vi "MQTT_Read_Published_Message.vi"(8 "error in (no error)":errorcluster, 11 "SSL_Connection":T2) -> (0 "error out":errorcluster, 1 "Message":string="MQIsdp", 2 "Topic Name":string="Topic", 3 "SSL_Connection":T2, 4 "MessageType":T1, 5 "Message ID":u16=1 format="%x")   [LabVIEW 2018, in "AWS_IoT.lvlib"]
doc: "This VI reads the last published message at the selected topic. It sends acknowledge information if required by the QoS level.\n\n© 2015 - daq.io, LLC - Peter Adelhardt"
uses:
  AWS_IoT.lvlib
  Controls/SSL_Connection.ctl
  Controls/MessageType.ctl
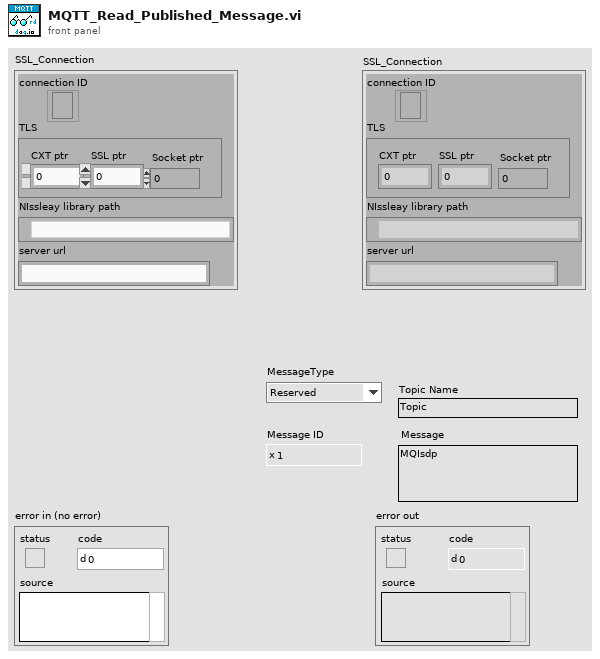
[diagram p1: front panel]
types:
  T1 = typedef "AWS_IoT.lvlib/MessageType.ctl" = enum32{"Reserved", "CONNECT", "CONNACK", "PUBLISH", "PUBACK", "PUBREC", "PUBREL", "PUBCOMP", "SUBSCRIBE", "SUBACK", "UNSUBSCRIBE", "UNSUBACK", "PINGREQ", "PINGRESP", "DISCONNECT", "Reserved2"}
  T2 = typedef "AWS_IoT.lvlib/SSL_Connection.ctl" = cluster{"connection ID":refnum<k5>, "TLS":cluster{"CXT ptr":i32, "SSL ptr":i32, "Socket ptr":i32}, "NIssleay library path":path, "server url":string}
  T3 = typedef "AWS_IoT.lvlib/QoS.ctl" = enum8{"At most once", "At least once", "Exactly once", "Reserved"}
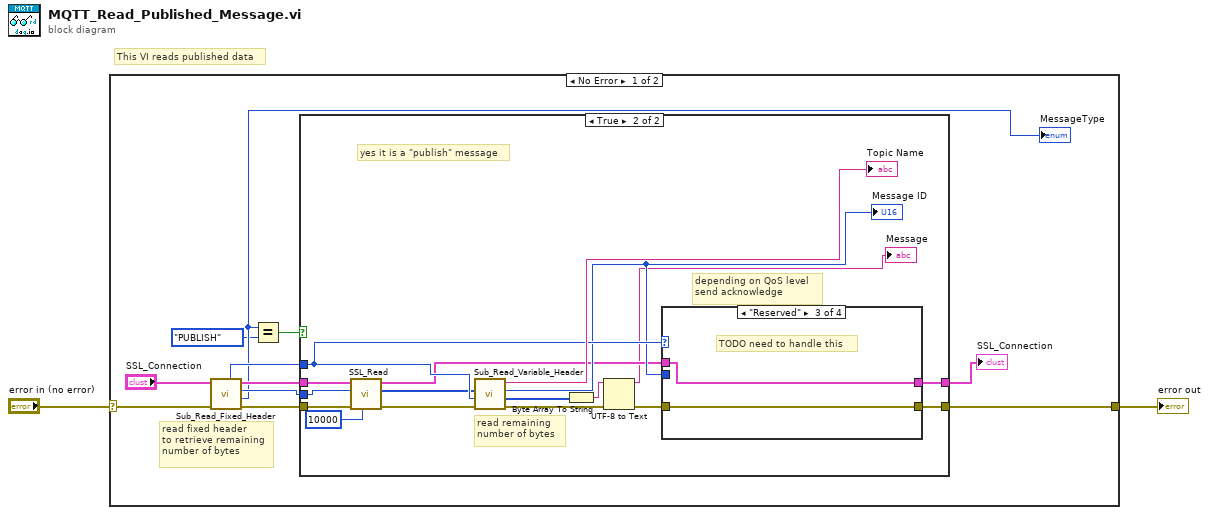
[diagram p0: block diagram]
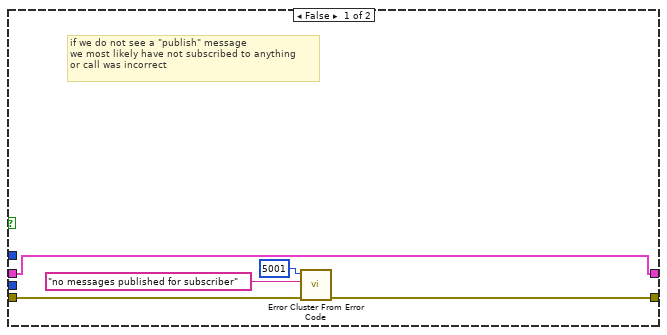
[diagram p2: hidden frame]
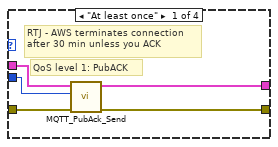
[diagram p3: hidden frame]
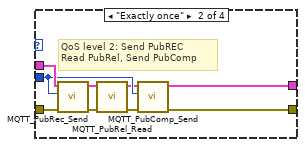
[diagram p4: hidden frame]
diagram:
  # "This VI reads published data"
  n1 = case shown="No Error" "error in (no error)" {
    selector: "error in (no error)" -> [w13 w54]
    tunnel: [w8 w54] -> w1
    frame No Error {
      # "read fixed header \nto retrieve remaining\nnumber of bytes"
      n2 = call "Sub_Read_Fixed_Header.vi"("error in (no error)"=w13, "SSL_Connection"="SSL_Connection") -> ("error out"=w10:errorcluster, "MessageType"=w7:T1, "Remaining Length"=w12:u32, "SSL_Connection"=w11:T2, "QoS Level"=w9:T3)  [unwired: 3 in, 2 out]
      "MessageType" <- w7
      n3 = Equal?(x=w7, y=MessageType."PUBLISH") -> (x = y?=w5:bool)
      n4 = case shown="True" w5 {
        tunnel: w12 -> [_ w34]
        tunnel: w11 -> [w14 w20]
        tunnel: w10 -> [w18 w33]
        tunnel: w9 -> [_ w31]
        tunnel: [w14 w28] -> w3
        tunnel: [w15 w27] -> w8
        frame False {
          # "if we do not see a \"publish\" message\nwe most likely have not subscribed to anything\nor call was incorrect"
          n5 = call <vilib>:"Error Cluster From Error Code.vi"("error in (no error)"=w18, "error message (\"\")"="no messages published for subscriber" ("error message (\"\")"), "error code (0)"=5001) -> ("error out"=w15:errorcluster)  [unwired: 6 in]
        }
        frame True {
          # "yes it is a \"publish\" message"
          # "depending on QoS level\nsend acknowledge"
          # "read remaining\nnumber of bytes"
          n6 = call "SSL_Read.vi"("timeout ms (5000)"=10000, "error in (no error)"=w33, "bytes to read"=w34, "SSL_Connection"=w20) -> ("error out"=w32:errorcluster, "data out"=w21:u8[], "SSL_Connection"=w29:T2)  [unwired: 4 in, 1 out]
          n7 = call "Sub_Read_Variable_Header.vi"("error in (no error)"=w32, "QoS"=w31, "Variable Header"=w21) -> ("error out"=w22:errorcluster, "remaining bytes"=w26:u8[], "Message ID"=w30:u16, "Topic Name"=→"Topic Name":string)  [unwired: 5 in]
          "Message ID" <- w30
          n8 = Byte Array To String(unsigned byte array=w26) -> (string=w25:string)
          n9 = UTF-8 to Text(8:w22, 11:w25) -> (0:w23:errorcluster, 3:→"Message":string)  [unwired: 1 in]
          n10 = case shown="\"Reserved\"" w31 {
            tunnel: w30 -> [w40 w45 _ _]
            tunnel: w23 -> [w39 w49 w50 w52]
            tunnel: w29 -> [w38 w48 w51 w53]
            tunnel: [w37 w47 w51 w53] -> w28
            tunnel: [w36 w46 w50 w52] -> w27
            frame "At least once" {
              # "RTJ - AWS terminates connection after 30 min unless you ACK"
              # "QoS level 1: PubACK"
              n11 = call "MQTT_PubAck_Send.vi"("error in (no error)"=w39, "Message ID"=w40, "SSL_Connection"=w38) -> ("error out"=w36:errorcluster, "SSL_Connection"=w37:T2)  [unwired: 6 in, 1 out]
            }
            frame "Exactly once" {
              # "QoS level 2: Send PubREC\nRead PubRel, Send PubComp"
              n12 = call "MQTT_PubRec_Send.vi"("error in (no error)"=w49, "Message ID"=w45, "SSL_Connection"=w48) -> ("error out"=w42:errorcluster, "SSL_Connection"=w41:T2)  [unwired: 6 in, 1 out]
              n13 = call "MQTT_PubRel_Read.vi"("error in (no error)"=w42, "SSL_Connection"=w41) -> ("error out"=w43:errorcluster, "SSL_Connection"=w44:T2)  [unwired: 7 in, 1 out]
              n14 = call "MQTT_PubComp_Send.vi"("error in (no error)"=w43, "Message ID"=w45, "SSL_Connection"=w44) -> ("error out"=w46:errorcluster, "SSL_Connection"=w47:T2)  [unwired: 6 in, 1 out]
            }
            frame "Reserved" {
              # "TODO need to handle this"
            }
            frame "At most once", Default {
              # "QoS level 0, no ACK"
            }
          }
        }
      }
      "SSL_Connection" <- w3
    }
    frame Error {
    }
  }
  "error out" <- w1
